vi "Fan_control.vi"() -> ()   [LabVIEW 2016]
uses:
  Typedef/MCU_addresses.ctl
  Typedef/Type_of_message_to_MCU.ctl
  Typedef/Type_of_request.ctl
panel:
  out "Byte array has been sent":u8[](array[numeric])
  in  "MCU Address to be sent":T1="G"
  in  "Slide":dbl(slide) scale=0.0..100.0
  in  "Play Button":bool
  in  "stop":bool
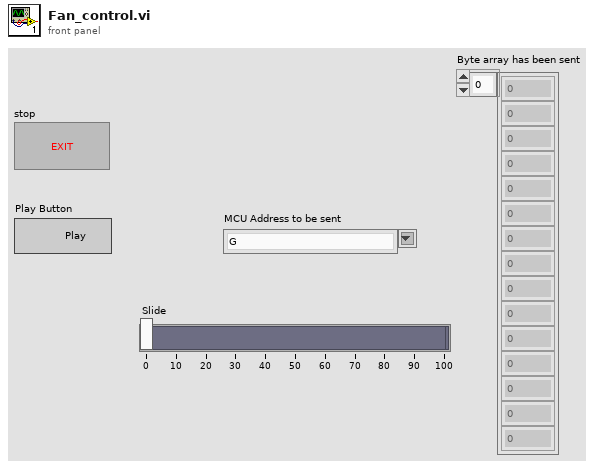
[diagram p1: front panel]
types:
  T1 = typedef "MCU_addresses.ctl" = string
  T2 = typedef "Type_of_message_to_MCU.ctl" = enum16{"Non", "Alarm", "Error", "Time and Date", "Status", "Request", "Command"}
  T3 = typedef "Type_of_request.ctl" = u8
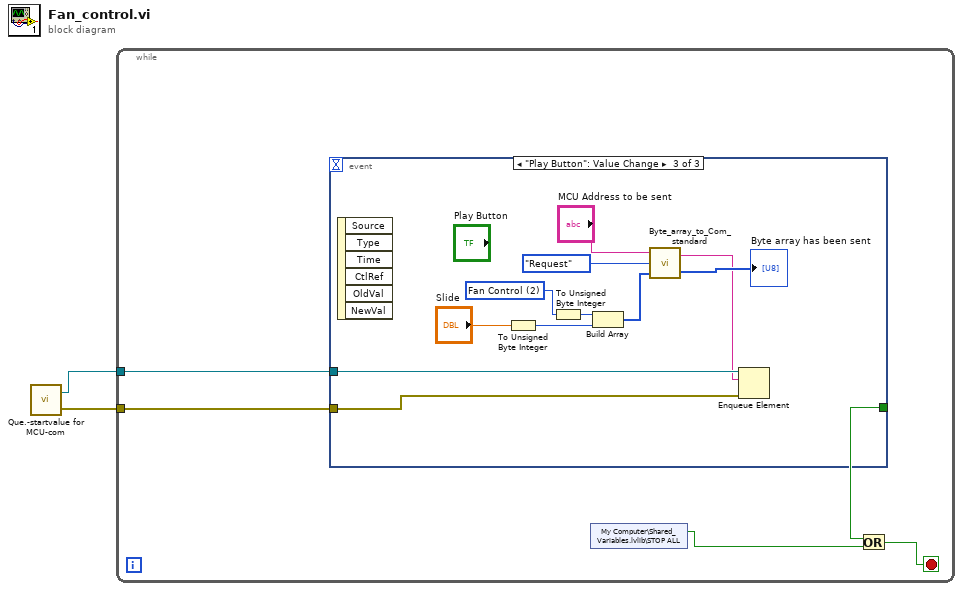
[diagram p0: block diagram]
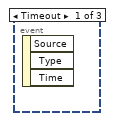
[diagram p2: hidden frame]
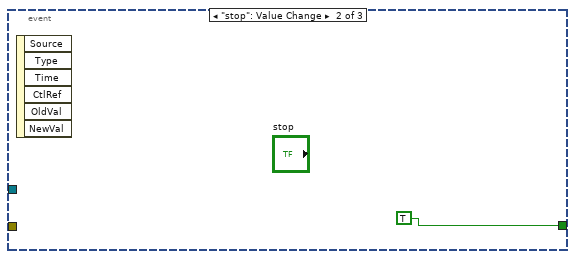
[diagram p3: hidden frame]
diagram:
  n1 = call "Que.-startvalue for MCU-com.vi"() -> ("error out"=w1:errorcluster, "queue out"=w2:refnum<queue>)  [unwired: 2 in]
  n2 = while {
    tunnel: w2 -> [w4]
    tunnel: w1 -> [w3]
    stop <- w6 stop-if-true
    n3 = event shown="[2] \"Play Button\": Value Change" {
      selector: _ -> [_ _ _]
      dyn-events: _ -> [_ _ _]
      timeout: _ -> [_ _ _]
      tunnel: [_ TRUE _] -> w7
      tunnel: w4 -> [_ _ w11]
      tunnel: w3 -> [_ _ w10]
      event Timeout {
        n4 = event-data() -> ()  [unwired: 1 in, 3 out]
      }
      event "stop": Value Change {
        n5 = event-data() -> ()  [unwired: 1 in, 6 out]
      }
      event "Play Button": Value Change {
        w12 = T3 2 items=["Unknown", "Neo-Pixel", "Fan Control", "Heat Control", "Display Text"] ("Ring")
        n6 = event-data() -> ()  [unwired: 1 in, 6 out]
        n7 = To Unsigned Byte Integer(number="Slide") -> (unsigned 8bit integer=w16:u8)
        n8 = To Unsigned Byte Integer(number=w12) -> (unsigned 8bit integer=w13:T3)
        n9 = Build Array(w13, w16) -> (w15:T3[])
        n10 = call "Byte_array_to_Com_standard.vi"("Payload  Byte to be sent"=w15, "Types of Data"=Type_of_message_to_MCU."Request", "MCU Address to be sent"="MCU Address to be sent") -> ("Byte array has been sent"=→"Byte array has been sent":u8[], "Converted Message"=w9:string)
        n11 = Enqueue Element(queue=w11, element=w9, error in (no error)=w10) -> ()  [unwired: 1 in, 3 out]
      }
    }
    n12 = shared-variable "My Computer\\Shared_Variables.lvlib\\STOP ALL"() -> (w5:bool)  [unwired: 1 in, 1 out]
    n13 = Or(x=w7, y=w5) -> (x .or. y?=w6:bool)
  }
